vi "Actor Core.vi"(8 "error in":errorcluster, 11 "1600 Card Actor in":refnum<class "1600 Card Actor.lvclass">) -> (0 "error out":errorcluster, 3 "Actor out":refnum<class "Actor.lvclass">)   [LabVIEW 2012, in "Universal Power Meter.lvlib" / "WT1600.lvlib" / "1600Card.lvlib" / "1600 Card Actor.lvclass"]
doc: "(<B>Filename</B>: Actor Framework.lvlib:Actor.lvclass:Actor Core.vi)\n\nReceives messages to the actor, reacts to them, and initiates any error handling that may shut the actor down.\n\nDescendant classes may override this VI to append parallel tasks for the actor to complete while it handles messages. Overrides use the Call Parent Method node."
uses:
  1600 Card Actor.lvclass
  <vilib>/ActorFramework/Actor/Actor.lvclass
  Display Panel/Power Meter Display/Power Meter Display.lvclass
  1600 Card Actor.lvclass/1600 Card Actor.ctl
  <vilib>/ActorFramework/Actor/Actor.lvclass/Actor.ctl
  <vilib>/ActorFramework/Message Enqueuer/Message Enqueuer.lvclass/Message Enqueuer.ctl
  Observer Pattern Actor Template/Observer/Observer.lvclass
  Display Panel/Power Meter Display Messages/Write Card# Msg/Write Card# Msg.lvclass/Write Card# Msg.ctl
  Display Panel/Power Meter Display Messages/Write Caption Ref Msg/Write Caption Ref Msg.lvclass/Write Caption Ref Msg.ctl
  Display Panel/Abstract Display Messages/Write time digit Msg/Write time digit Msg.lvclass/Write time digit Msg.ctl
  Data Logger/Data Logger Messages/Write Time Out Ref Msg/Write Time Out Ref Msg.lvclass/Write Time Out Ref Msg.ctl
  Data Logger/Data Logger Messages/Write Signal Ref Msg/Write Signal Ref Msg.lvclass/Write Signal Ref Msg.ctl
  Display Panel/Power Meter Display Messages/Write Voltage Msg/Write Voltage Msg.lvclass/Write Voltage Msg.ctl
  Display Panel/Power Meter Display Messages/Write Curr. Ref Msg/Write Curr. Ref Msg.lvclass/Write Curr. Ref Msg.ctl
  Display Panel/Power Meter Display Messages/Write Freq. Ref Msg/Write Freq. Ref Msg.lvclass/Write Freq. Ref Msg.ctl
  Display Panel/Power Meter Display Messages/Write Pow. Ref  Msg/Write Pow. Ref  Msg.lvclass/Write Pow. Ref  Msg.ctl
  Display Panel/Power Meter Display Messages/Write W-Hrs. Ref  Msg/Write W-Hrs. Ref  Msg.lvclass/Write W-Hrs. Ref  Msg.ctl
  Display Panel/Power Meter Display Messages/Write Blink Msg/Write Blink Msg.lvclass/Write Blink Msg.ctl
  WT1600/WT1600 Messages/Integration Start Stop Msg/Integration Start Stop Msg.lvclass/Integration Start Stop Msg.ctl
  <vilib>/ActorFramework/Message Enqueuer/Init from Existing Queue.vi
  <vilib>/ActorFramework/Message Enqueuer/Enqueue.vi
  <vilib>/ActorFramework/Message Priority Queue/Priority Enqueue.vi
  <vilib>/ActorFramework/Message Enqueuer/Message Enqueuer.lvclass
  <vilib>/ActorFramework/Stop Msg/Stop Msg.lvclass
  Display Panel/Power Meter Display Messages/Write Card# Msg/Write Card# Msg.lvclass
  Display Panel/Power Meter Display Messages/Write Caption Ref Msg/Write Caption Ref Msg.lvclass
  Display Panel/Abstract Display Messages/Write time digit Msg/Write time digit Msg.lvclass
  Data Logger/Data Logger Messages/Write Time Out Ref Msg/Write Time Out Ref Msg.lvclass
  Data Logger/Data Logger Messages/Write Signal Ref Msg/Write Signal Ref Msg.lvclass
  Display Panel/Power Meter Display Messages/Write Voltage Msg/Write Voltage Msg.lvclass
  Display Panel/Power Meter Display Messages/Write Curr. Ref Msg/Write Curr. Ref Msg.lvclass
  Display Panel/Power Meter Display Messages/Write Freq. Ref Msg/Write Freq. Ref Msg.lvclass
  Display Panel/Power Meter Display Messages/Write Pow. Ref  Msg/Write Pow. Ref  Msg.lvclass
  Display Panel/Power Meter Display Messages/Write W-Hrs. Ref  Msg/Write W-Hrs. Ref  Msg.lvclass
  Display Panel/Power Meter Display Messages/Write Blink Msg/Write Blink Msg.lvclass
  WT1600/WT1600 Messages/Integration Start Stop Msg/Integration Start Stop Msg.lvclass
  Generic Instrument/Generic Instrument.lvclass
  Data Logger/Data Logger.lvclass
panel:
  out "Start blinking":bool=TRUE
  in  "Stop bit":bool
  in  "Display Panel.lvlib:Power Meter Display.lvclass":refnum<class "Power Meter Display.lvclass">
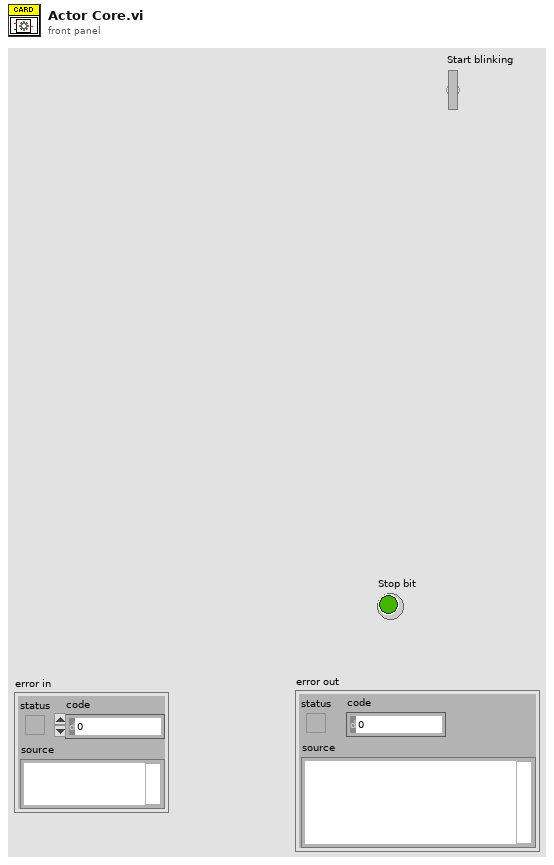
[diagram p1: front panel]
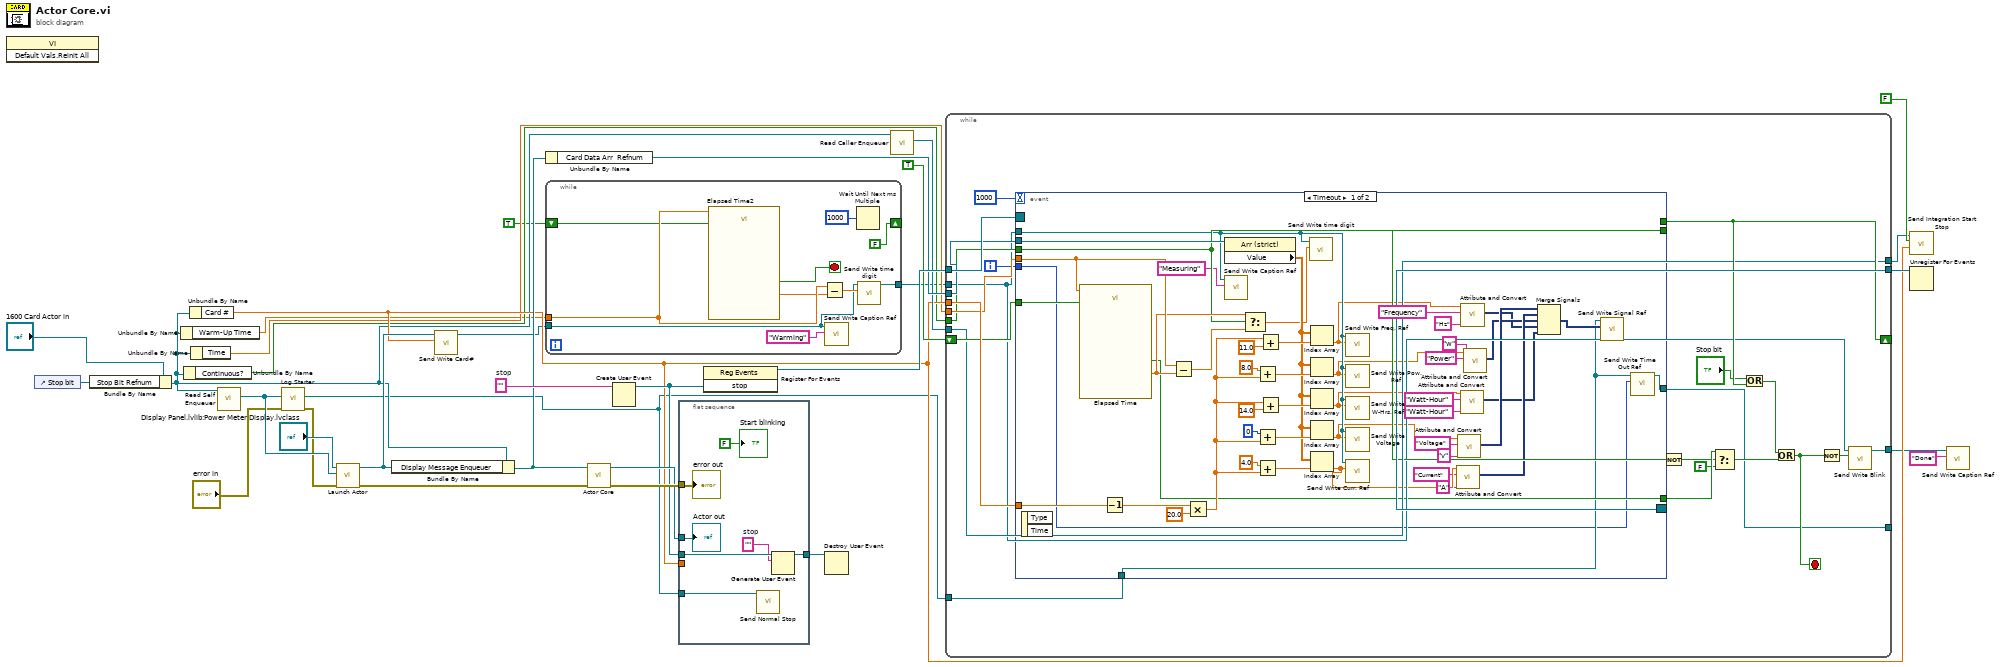
[diagram p0: block diagram]
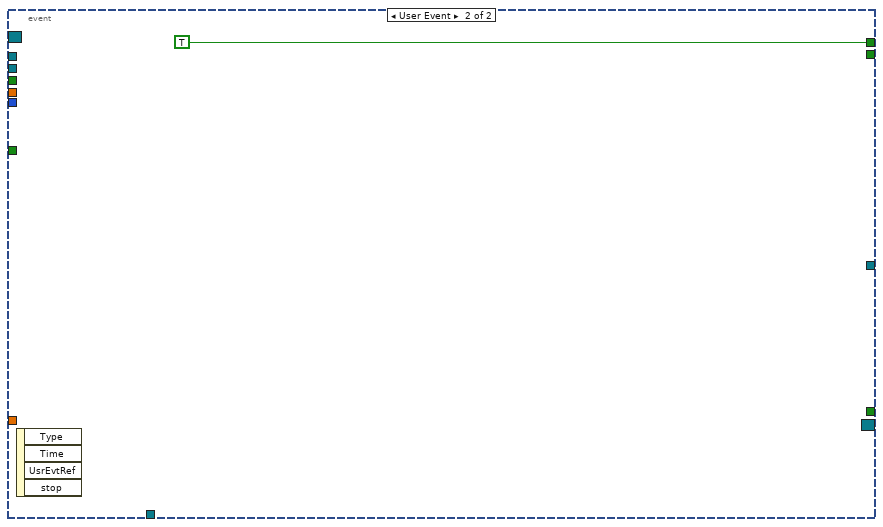
[diagram p2: hidden frame]
diagram:
  w27 = ""  # stop
  n1 = invoke class="VI" method="Default Vals.Reinit All"() -> ()  [unwired: 3 in, 3 out]
  n2 = control-ref of="Stop bit"() -> (w18:refnum<vi>)
  n3 = Bundle By Name(cluster="1600 Card Actor in", "Stop Bit Refnum"=w18) -> (w11:refnum<class "1600 Card Actor.lvclass">)
  n4 = Unbundle By Name(w11) -> ("Warm-Up Time"=w10:dbl)
  n5 = Unbundle By Name(w11) -> ("Continuous?"=w13:bool)
  n6 = Unbundle By Name(w11) -> ("Card #"=w14:dbl)
  n7 = Unbundle By Name(w11) -> ("Time"=w12:dbl)
  n8 = call <vilib>:"Read Self Enqueuer.vi"("Actor"=w11) -> ("Self Enqueuer"=w4:refnum<class "Message Enqueuer.lvclass">)  [unwired: 10 in]
  n9 = call "Log Starter.vi"("error in"="error in", "Actor-to-Caller Enqueuer"=w4) -> ("error in"=w1:errorcluster, "Caller-To-Actor Enqueuer"=w3:refnum<class "Message Enqueuer.lvclass">)  [unwired: 8 in]
  n10 = call <vilib>:"Launch Actor.vi"("error in (no error)"=w1, "Actor-to-Caller Enqueuer"=w4, "Actor"="Display Panel.lvlib:Power Meter Display.lvclass") -> ("error out"=w30:errorcluster, "Caller-To-Actor Enqueuer"=w28:refnum<class "Message Enqueuer.lvclass">)  [unwired: 7 in]
  n11 = Bundle By Name(cluster=w11, "Display Message Enqueuer"=w28) -> (w21:refnum<class "1600 Card Actor.lvclass">)
  n12 = call "Send Write Card#.vi"("Card#"=w14, "Message Enqueuer"=w28) -> ("Message Enqueuer out"=w9:refnum<class "Message Enqueuer.lvclass">)  [unwired: 8 in, 1 out]
  n13 = Unbundle By Name(w21) -> ("Card Data Arr  Refnum"=w20:refnum<vi>)
  n14 = while {
    tunnel: w10 -> [w42]
    tunnel: [w40] -> w8
    tunnel: w9 -> [w33]
    shift-right: [FALSE] -> _
    shift-left: TRUE -> [w39]
    stop <- w37 stop-if-true
    n15 = call "Elapsed Time2"("Time Target (s)"=w42, "Reset"=w39) -> ("Elapsed Time (s)"=w41:dbl, "Time has Elapsed"=w37:bool)  [unwired: 10 in, 6 out]
    n16 = Subtract(x=w42, y=w41) -> (x-y=w36:dbl)
    n17 = call "Send Write Caption Ref.vi"("Caption"="Warming", "Message Enqueuer"=w33) -> ()  [unwired: 8 in, 2 out]
    n18 = Wait Until Next ms Multiple(millisecond multiple=u32 1000) -> ()  [unwired: 1 out]
    n19 = call "Send Write time digit.vi"("Time"=w36, "Message Enqueuer"=w33) -> ("Message Enqueuer out"=w40:refnum<class "Message Enqueuer.lvclass">)  [unwired: 8 in, 1 out]
  }
  n20 = call-parent "Actor Core.vi"("error in"=w30, "Actor in"=w21) -> ("error out"=w32:errorcluster, "Actor out"=w31:refnum<class "Actor.lvclass">)  [unwired: 8 in]
  n21 = Create User Event(user event datatype=w27) -> (user event=w24:refnum<user-event>)  [unwired: 1 in, 1 out]
  n22 = flat-sequence {
    tunnel: w32 -> [w49]
    tunnel: w31 -> [w48]
    tunnel: w24 -> [w47]
    tunnel: [w45] -> w23
    tunnel: w14 -> [_]
    tunnel: w3 -> [w43]
    frame #0 {
      w46 = ""  # stop
      n23 = call <vilib>:"Send Normal Stop.vi"("Message Enqueuer"=w43) -> ()  [unwired: 10 in, 1 out]
      n24 = Generate User Event(user event=w47, event data cluster=w46) -> (user event out=w45:refnum<user-event>)  [unwired: 1 in, 1 out]
      "error out" <- w49
      "Actor out" <- w48
      "Start blinking" <- FALSE ("stop blinking")
    }
  }
  n25 = register-events(w24) -> (reference out=w26:refnum<event-registration>)  [unwired: 2 in, 1 out]
  n26 = Destroy User Event(user event=w23) -> ()  [unwired: 1 in, 1 out]
  n27 = call <vilib>:"Read Caller Enqueuer.vi"("Actor"=w11) -> ("Caller Enqueuer"=w17:refnum<class "Message Enqueuer.lvclass">)  [unwired: 10 in]
  n28 = while {
    tunnel: w8 -> [w56]
    tunnel: w26 -> [w72]
    tunnel: [w71] -> w25
    tunnel: w14 -> [w70]
    shift-right: [w67] -> _
    shift-left: TRUE -> [w69]
    tunnel: w20 -> [w68]
    tunnel: w17 -> [w65]
    tunnel: [w65] -> w15
    tunnel: w13 -> [w63]
    tunnel: w12 -> [w64]
    tunnel: [w53] -> w6
    tunnel: w3 -> [w52]
    tunnel: [w50] -> _
    i -> [w51]
    stop <- w55 stop-if-true
    n29 = event shown="[0] Timeout" {
      selector: w72 -> [_ _]
      dyn-events: [_ _] -> w71
      timeout: u32 1000 ("millisecond multiple") -> [_ _]
      tunnel: w56 -> [w99 _]
      tunnel: [_ TRUE ("Stop Button")] -> w67
      tunnel: w70 -> [w122 _]
      tunnel: w69 -> [w108 _]
      tunnel: w68 -> [w106 _]
      tunnel: w64 -> [w104 _]
      tunnel: w63 -> [w102 _]
      tunnel: [w102 _] -> w59
      tunnel: [w101 _] -> w61
      tunnel: w52 -> [w76 _]
      tunnel: w51 -> [w75 _]
      tunnel: [w74 _] -> w50
      event Timeout {
        n30 = event-data() -> ()  [unwired: 1 in, 2 out]
        n31 = call "Elapsed Time"("Time Target (s)"=w104, "Reset"=w108) -> ("Elapsed Time (s)"=w103:dbl, "Time has Elapsed"=w101:bool)  [unwired: 10 in, 6 out]
        n32 = Decrement(x=w122) -> (x-1=w121:dbl)
        n33 = Subtract(x=w104, y=w103) -> (x-y=w105:dbl)
        n34 = Multiply(x=w121, y=20.0) -> (x*y=w112:dbl)
        n35 = property class="Arr (strict)"(reference=w106) -> ("Value"=w107:dbl[])  [unwired: 1 in, 2 out]
        n36 = call "Send Write Caption Ref.vi"("Caption"="Measuring", "Message Enqueuer"=w99) -> ()  [unwired: 8 in, 2 out]
        n37 = Select(t=w103, s=w102, f=w105) -> (s? t:f=w100:dbl)
        n38 = Add(x=8.0, y=w112) -> (x+y=w114:dbl)
        n39 = Add(x=0 ("index"), y=w112) -> (x+y=w117:dbl)
        n40 = Add(x=4.0, y=w112) -> (x+y=w116:dbl)
        n41 = Add(x=w112, y=11.0) -> (x+y=w110:dbl)
        n42 = Add(x=w112, y=14.0) -> (x+y=w109:dbl)
        n43 = call "Send Write time digit.vi"("Time"=w100, "Message Enqueuer"=w99) -> ()  [unwired: 8 in, 2 out]
        n44 = Index Array(array=w107, index=w110) -> (element=w97:dbl)
        n45 = Index Array(array=w107, index=w114) -> (element=w94:dbl)
        n46 = Index Array(array=w107, index=w109) -> (element=w91:dbl)
        n47 = Index Array(array=w107, index=w117) -> (element=w88:dbl)
        n48 = Index Array(array=w107, index=w116) -> (element=w85:dbl)
        n49 = call "Send Write Freq. Ref.vi"("Freq. Ref"=w97, "Message Enqueuer"=w99) -> ()  [unwired: 8 in, 2 out]
        n50 = call "Send Write Pow. Ref .vi"("Pow. Ref"=w94, "Message Enqueuer"=w99) -> ()  [unwired: 8 in, 2 out]
        n51 = call "Send Write W-Hrs. Ref .vi"("W-Hrs. Ref"=w91, "Message Enqueuer"=w99) -> ()  [unwired: 8 in, 2 out]
        n52 = call "Send Write Voltage.vi"("Voltage"=w88, "Message Enqueuer"=w99) -> ()  [unwired: 8 in, 2 out]
        n53 = call "Send Write Curr. Ref.vi"("Curr. Ref"=w85, "Message Enqueuer"=w99) -> ()  [unwired: 8 in, 2 out]
        n54 = call "Attribute and Convert.vi"("Unit"="A", "Signal Name"="Current", "Number in"=w85) -> ("Dynamic Signal Out"=w81:dynamicdata)  [unwired: 8 in]
        n55 = call "Attribute and Convert.vi"("Unit"="v", "Signal Name"="Voltage", "Number in"=w88) -> ("Dynamic Signal Out"=w82:dynamicdata)  [unwired: 8 in]
        n56 = call "Attribute and Convert.vi"("Unit"="Watt-Hour", "Signal Name"="Watt-Hour", "Number in"=w91) -> ("Dynamic Signal Out"=w78:dynamicdata)  [unwired: 8 in]
        n57 = call "Attribute and Convert.vi"("Unit"="Hz", "Signal Name"="Frequency", "Number in"=w97) -> ("Dynamic Signal Out"=w79:dynamicdata)  [unwired: 8 in]
        n58 = call "Attribute and Convert.vi"("Unit"="w", "Signal Name"="Power", "Number in"=w94) -> ("Dynamic Signal Out"=w80:dynamicdata)  [unwired: 8 in]
        n59 = Merge Signals(w82, w81, w80, w79, w78) -> (w77:dynamicdata)
        n60 = call "Send Write Signal Ref.vi"("Waveform Graph"=w77, "Message Enqueuer"=w76) -> ()  [unwired: 8 in, 2 out]
        n61 = call "Send Write Time Out Ref.vi"("Numeric"=w75, "Message Enqueuer"=w76) -> ("Message Enqueuer out"=w74:refnum<class "Message Enqueuer.lvclass">)  [unwired: 8 in, 1 out]
      }
      event User Event {
        n62 = event-data() -> ()  [unwired: 1 in, 4 out]
      }
    }
    n63 = Not(x=w59) -> (.not. x?=w58:bool)
    n64 = Select(t=w61, s=w58, f=FALSE) -> (s? t:f=w60:bool)
    n65 = Or(x="Stop bit", y=w67) -> (x .or. y?=w62:bool)
    n66 = Or(x=w62, y=w60) -> (x .or. y?=w55:bool)
    n67 = Not(x=w55) -> (.not. x?=w54:bool)
    n68 = call "Send Write Blink.vi"("Blink? Ref"=w54, "Message Enqueuer"=w56) -> ("Message Enqueuer out"=w53:refnum<class "Message Enqueuer.lvclass">)  [unwired: 8 in, 1 out]
  }
  n69 = call "Send Integration Start Stop.vi"("Element (All: 0)"=w14, "Start/Stop (F: Stop)"=FALSE, "Message Enqueuer"=w15) -> ()  [unwired: 7 in, 2 out]
  n70 = Unregister For Events(event registration refnum=w25) -> ()  [unwired: 1 in, 1 out]
  n71 = call "Send Write Caption Ref.vi"("Caption"="Done", "Message Enqueuer"=w6) -> ()  [unwired: 8 in, 2 out]
